vi "Read_camCalOffset.vi"() -> (3 "cam_CAL_OFFSET":bool)   [LabVIEW 2023, in "Cam Data.lvlib"]
uses:
  Cam Data.lvlib
panel:
  out "?":string
  out "Status":string="No Error"
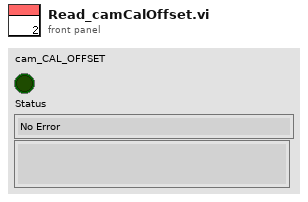
[diagram p1: front panel]
types:
  T1 = cluster{"Address IP":string, "Rack":i32, "Slot ":i32, "DB Number":i32, "Start":i32, "Amount":i32}
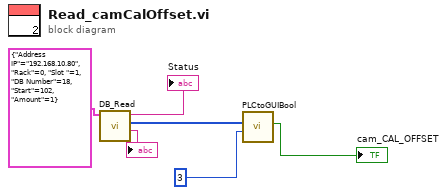
[diagram p0: block diagram]
diagram:
  n1 = call "DB_Read.vi"("Input Params"=T1 {"Address IP"="192.168.10.80", "Rack"=0, "Slot "=1, "DB Number"=18, "Start"=102, "Amount"=1}) -> (1:→"?":string, "Data"=w5:u8[], "Status"=→"Status":string)  [unwired: 8 in]
  n2 = call "PLCtoGUIBool.vi"("SubOffset"=u16 3, "DB Input Vals"=w5) -> ("element"=→"cam_CAL_OFFSET":bool)  [unwired: 9 in]
